vi "Input to Waveform Chart.vi"(9 "TagArray":refnum<class "Tag.lvclass">[](array[class]), 11 "output array":T1(array[cluster])) -> (1 "Measured error margin chart":dbl[][](graph))   [LabVIEW 2014]
uses:
  Tag.lvclass
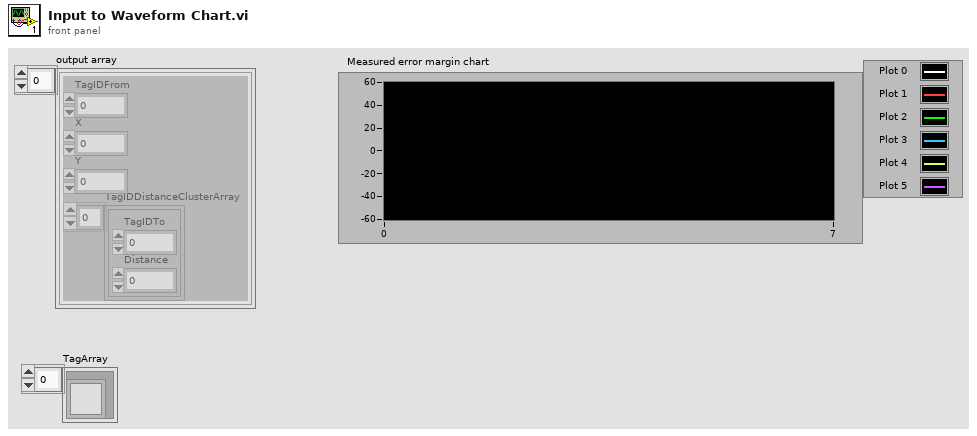
[diagram p1: front panel]
types:
  T1 = cluster{"TagIDFrom":dbl, "X":dbl, "Y":dbl, "TagIDDistanceClusterArray":cluster{"TagIDTo":dbl, "Distance":dbl}[]}[]
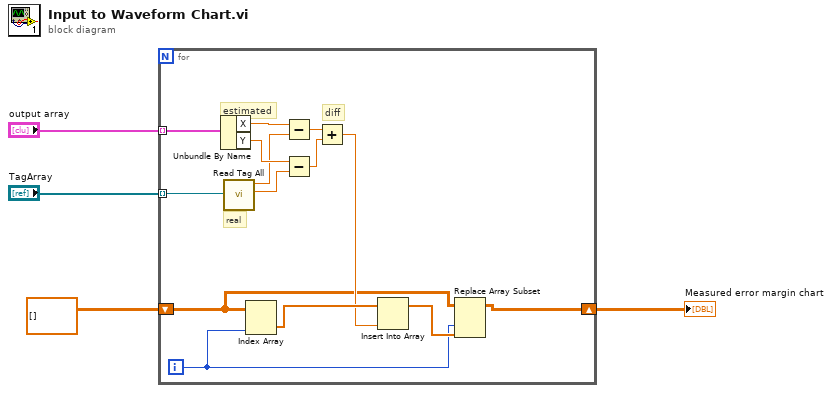
[diagram p0: block diagram]
diagram:
  n1 = for {
    tunnel: "output array" -> [w12] mode=indexing
    tunnel: "TagArray" -> [w11] mode=indexing
    shift-right: [w6] -> w2
    shift-left: dbl[][] [] -> [w8]
    i -> [w5]
    # "diff"
    # "real"
    # "estimated"
    n2 = Unbundle By Name ("estimated xy values")(w12) -> ("X"=w14:dbl, "Y"=w18:dbl)
    n3 = call "Read Tag All.vi"("Tag.lvclass"=w11) -> ("TagY"=w17:dbl, "TagX"=w13:dbl)  [unwired: 5 in, 4 out]
    n4 = Index Array(array=w8, index (col)=w5) -> (element=w10:dbl[])  [unwired: 1 in]
    n5 = Subtract(x=w14, y=w13) -> (x-y=w16:dbl)
    n6 = Subtract(x=w18, y=w17) -> (x-y=w15:dbl)
    n7 = Add(x=w16, y=w15) -> (x+y=w9:dbl)
    n8 = Insert Into Array(array=w10, new element=w9) -> (w7:dbl[])  [unwired: 1 in]
    n9 = Replace Array Subset(array=w8, new element=w7, index (col)=w5) -> (w6:dbl[][])  [unwired: 1 in]
  }
  "Measured error margin chart" <- w2
